vi "GetParam.vi"(1 "IniParams":T1, 5 "error in (no error)":errorcluster) -> (15 "Value":string, 17 "Array":cluster{string, "Value":string}[](array[cluster]), 19 "error out":errorcluster)   [LabVIEW 2014, in "UmlEditor.lvclass"]
uses:
  <resource>/Framework/Providers/Open_GDS/UML/UmlEditor_class/UmlEditor.lvclass
  <resource>/Framework/Providers/Open_GDS/UML/UmlEditor_class/IniParamsType.ctl
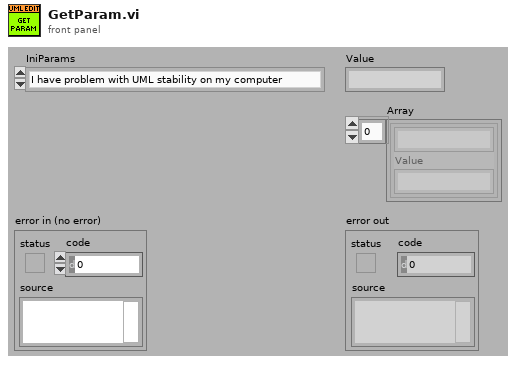
[diagram p1: front panel]
types:
  T1 = typedef "UmlEditor.lvclass/IniParamsType.ctl" = enum16{"I have problem with UML stability on my computer"}
  T2 = typedef "UmlEditor.lvclass/ObjectAttributes.ctl" = cluster{"ListeningQueueIn":refnum<queue>, "Event":refnum<user-event>, "UseProjectFolderAsBasePath":bool, "TypeSyncOption":bool, "Attr":string[], "ToolTip":cluster{"ToolTipOpen":bool, "LastToolTip":i32}, "ClassesToIgnore":string[], "UndoSize":i32, "OpenLastSavedFileWhenStarting":bool, "SyncOption":T3, "SyncTime(s)":i32, "Params":cluster{"IniParams":T1, "Value":string}[]}
  T3 = typedef "UMLEditor_SyncOptions.ctl" = cluster{"IgnoreInstrLib":bool, "IgnoreUserLib":bool, "IgnoreViLib":bool}
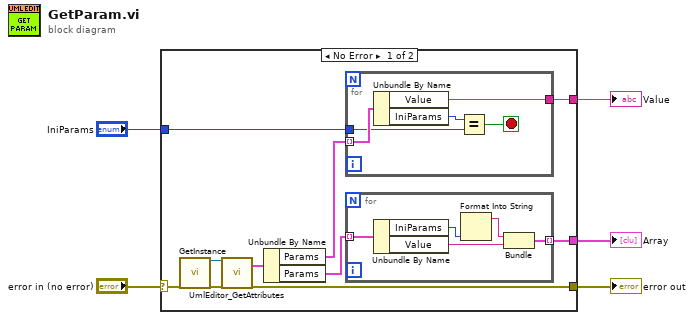
[diagram p0: block diagram]
diagram:
  n1 = case shown="No Error" "error in (no error)" {
    selector: "error in (no error)" -> [w13 w26]
    tunnel: [w12 w26] -> w4
    tunnel: "IniParams" -> [w10 _]
    tunnel: [w9 _] -> w2
    tunnel: [w7 _] -> w1
    frame No Error {
      n2 = call <resource>:"GetInstance.vi"("error in (no error)"=w13) -> ("reference out"=w15:refnum<class "UmlEditor.lvclass">, "error out"=w14:errorcluster)  [unwired: 17 out]
      n3 = call <resource>:"UmlEditor_GetAttributes.vi"("reference in"=w15, "error in (no error)"=w14) -> ("Data"=w6:T2, "error out"=w12:errorcluster)  [unwired: 14 in, 2 out]
      n4 = Unbundle By Name(w6) -> ("Params"=w11:cluster{"IniParams":T1, "Value":string}[], "Params"=w8:cluster{"IniParams":T1, "Value":string}[])
      n5 = for {
        tunnel: w11 -> [w25] mode=indexing
        tunnel: w10 -> [w23]
        tunnel: [w21] -> w9
        stop <- w22 stop-if-true
        n6 = Unbundle By Name(w25) -> ("Value"=w21:string, "IniParams"=w24:T1)
        n7 = Equal?(x=w24, y=w23) -> (x = y?=w22:bool)
      }
      n8 = for {
        tunnel: w8 -> [w20] mode=indexing
        tunnel: [w17] -> w7 mode=indexing
        n9 = Unbundle By Name(w20) -> ("IniParams"=w16:T1, "Value"=w18:string)
        n10 = Format Into String(w16) -> (resulting string=w19:string)  [unwired: 3 in, 1 out]
        n11 = Bundle(w19, "Value"=w18) -> (w17:cluster{string, "Value":string})  [unwired: 1 in]
      }
    }
    frame Error {
    }
  }
  "error out" <- w4
  "Value" <- w2
  "Array" <- w1
